vi "Force Destroy Enqueuer.vi"(8 "error in (no error)":errorcluster, 11 "QDMH in":refnum<class "QDMH.lvclass">) -> (0 "error out":errorcluster, 3 "QDMH out":refnum<class "QDMH.lvclass">)   [LabVIEW 2023, in "QDMH.lvlib" / "QDMH.lvclass"]
doc: "This tool is designed to destroy all named queue references. \n\nThis completely eliminates the queue and must be called by the master queue administrator."
uses:
  Library/QDMH.lvclass
  Library/QDMH.lvclass/QDMH.ctl
  Custom Controls/Message.ctl
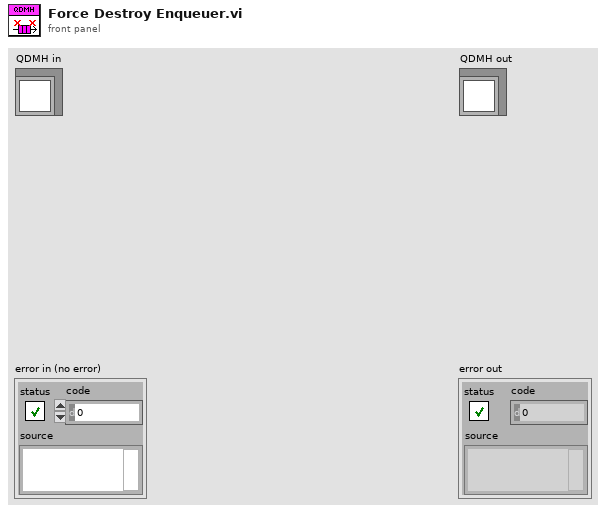
[diagram p1: front panel]
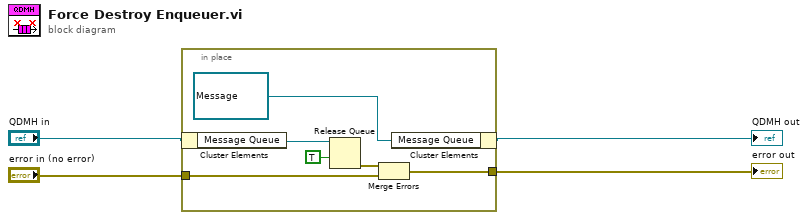
[diagram p0: block diagram]
diagram:
  n1 = in-place {
    in-place-border: "error in (no error)" -> [w7]
    in-place-border: [w6] -> w2
    n2 = in-place-cluster #1("QDMH in") -> ("Message Queue"=w10:refnum<queue>)
    n3 = Release Queue(queue=w10, force destroy? (F)=TRUE) -> (error out=w8:errorcluster)  [unwired: 1 in, 2 out]
    n4 = Merge Errors(w8, w7) -> (w6:errorcluster)
    n5 = in-place-cluster #1("Message Queue"=refnum<queue> refnum) -> (→"QDMH out":refnum<class "QDMH.lvclass">)
  }
  "error out" <- w2
